vi "TC to PGSQL.vi"(8 "error in (no error)":errorcluster, 11 "TC Cluster":T1) -> (0 "error out":errorcluster)   [LabVIEW 2016]
uses:
  Typedefs/TC-cluster.ctl
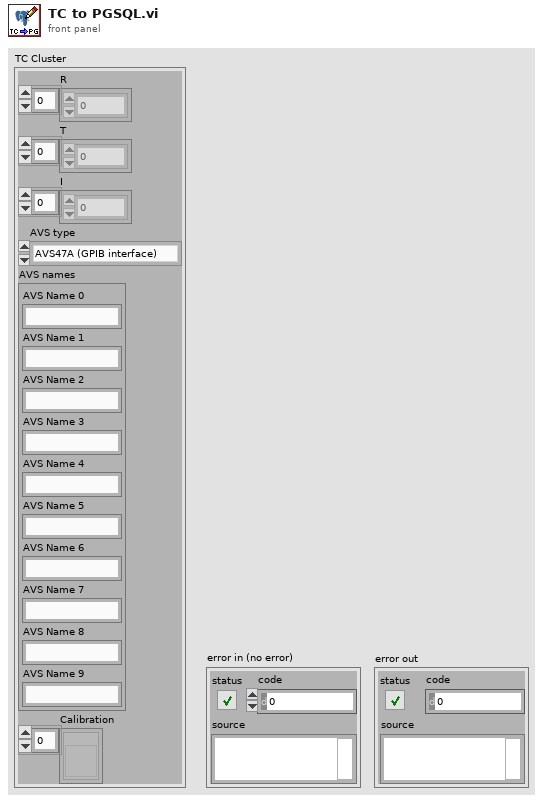
[diagram p1: front panel]
types:
  T1 = typedef "TC-cluster.ctl" = cluster{"R":dbl[], "T":dbl[], "I":dbl[], "AVS type":enum16{"AVS47A (GPIB interface)", "AVS47B (RS232 interface)", "AVS48", "AVS Emulation", "Impedance Bridge", "Disabled"}, "AVS names":cluster{"AVS Name 0":string, "AVS Name 1":string, "AVS Name 2":string, "AVS Name 3":string, "AVS Name 4":string, "AVS Name 5":string, "AVS Name 6":string, "AVS Name 7":string, "AVS Name 8":string, "AVS Name 9":string}, "Calibration":refnum<vi>[]}
  T2 = enum16{"AVS47A (GPIB interface)", "AVS47B (RS232 interface)", "AVS48", "AVS Emulation", "Impedance Bridge", "Disabled"}
  T3 = cluster{"AVS Name 0":string, "AVS Name 1":string, "AVS Name 2":string, "AVS Name 3":string, "AVS Name 4":string, "AVS Name 5":string, "AVS Name 6":string, "AVS Name 7":string, "AVS Name 8":string, "AVS Name 9":string}
  T4 = enum16{"CF", "CF_Z_Bridge", "MNK", "MNK_Z_Bridge"}
  T5 = cluster{"[0]":string, "[1]":string, "[2]":string, "[3]":string, "[4]":string, "[5]":string, "[6]":string, "[7]":string, "[8]":string, "[9]":string}
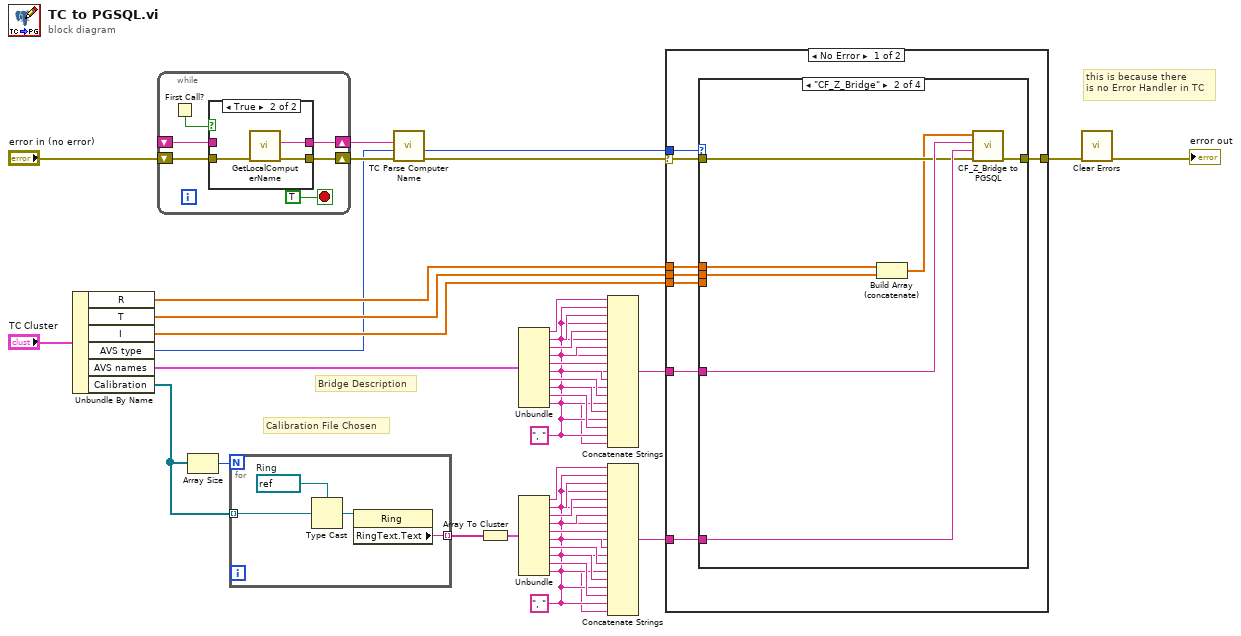
[diagram p0: block diagram]
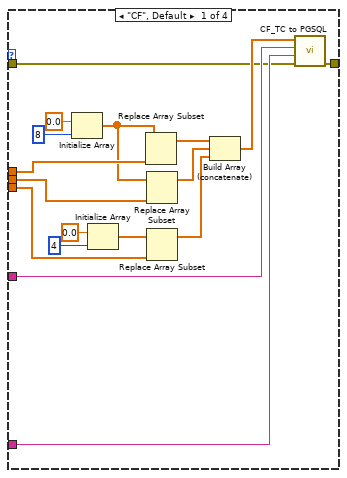
[diagram p3: hidden frame]
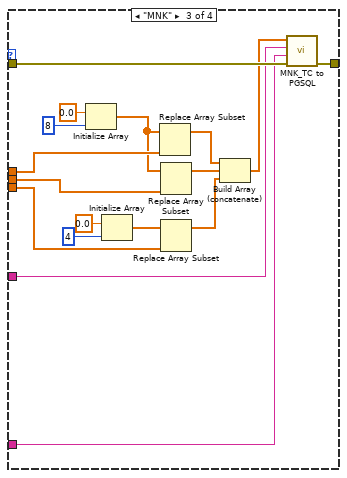
[diagram p4: hidden frame]
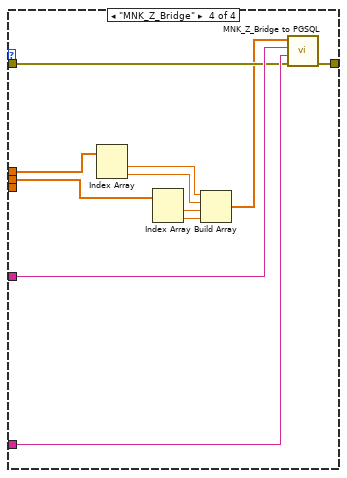
[diagram p5: hidden frame]
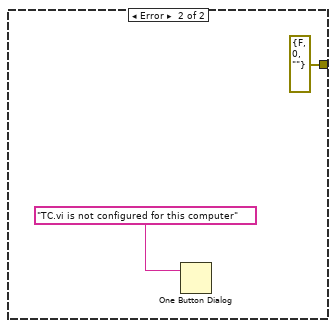
[diagram p6: hidden frame]
diagram:
  w18 = ", " ("string")
  w32 = ", " ("string")
  # "this is because there\nis no Error Handler in TC"
  # "Bridge Description"
  # "Calibration File Chosen"
  n1 = Unbundle By Name("TC Cluster") -> ("R"=w9:dbl[], "T"=w8:dbl[], "I"=w7:dbl[], "AVS type"=w4:T2, "AVS names"=w6:T3, "Calibration"=w5:refnum<vi>[])
  n2 = while {
    shift-right: [w46] -> w12
    shift-left: "error in (no error)" -> [w43]
    shift-right: [w47] -> w3
    shift-left: _ -> [w42]
    stop <- TRUE stop-if-true
    n3 = First Call?() -> (First Call?: T/F=w45:bool)
    n4 = case shown="True" w45 {
      tunnel: [w49 w52] -> w47
      tunnel: [w48 w51] -> w46
      tunnel: w43 -> [w48 w50]
      tunnel: w42 -> [w49 _]
      frame False {
      }
      frame True {
        n5 = call "GetLocalComputerName.vi"("error in (no error)"=w50) -> ("error out"=w51:errorcluster, "Name"=w52:string)  [unwired: 8 in, 1 out]
      }
    }
  }
  n6 = Array Size(array=w5) -> (size(s)=w29:i32)
  n7 = for {
    N: w29 -> [_]
    tunnel: w5 -> [w56] mode=indexing
    tunnel: [w53] -> w28 mode=indexing
    w55 = refnum<vi> refnum  # Ring
    n8 = Type Cast(type=w55, x=w56) -> (*(type *) &x=w54:refnum<vi>)
    n9 = property class="Ring"(reference=w54) -> ("RingText.Text"=w53:string)  [unwired: 1 in, 2 out]
  }
  n10 = call "TC Parse Computer Name.vi"("error in (no error)"=w12, "AVS type"=w4, "computer name"=w3) -> ("error out"=w13:errorcluster, "AVS Type"=w14:T4)  [unwired: 7 in]
  n11 = Array To Cluster(array=w28) -> (cluster=w16:T5)
  n12 = Unbundle(w6) -> ("AVS Name 0"=w41:string, "AVS Name 1"=w40:string, "AVS Name 2"=w39:string, "AVS Name 3"=w38:string, "AVS Name 4"=w37:string, "AVS Name 5"=w36:string, "AVS Name 6"=w35:string, "AVS Name 7"=w34:string, "AVS Name 8"=w33:string, "AVS Name 9"=w31:string)
  n13 = Unbundle(w16) -> ("[0]"=w27:string, "[1]"=w26:string, "[2]"=w25:string, "[3]"=w24:string, "[4]"=w23:string, "[5]"=w22:string, "[6]"=w21:string, "[7]"=w20:string, "[8]"=w19:string, "[9]"=w17:string)
  n14 = Concatenate Strings(w41, w32, w40, w32, w39, w32, w38, w32, w37, w32, w36, w32, w35, w32, w34, w32, w33, w32, w31) -> (w30:string)
  n15 = Concatenate Strings(w27, w18, w26, w18, w25, w18, w24, w18, w23, w18, w22, w18, w21, w18, w20, w18, w19, w18, w17) -> (w15:string)
  n16 = case shown="No Error" w13 {
    selector: w13 -> [w58 _]
    tunnel: w30 -> [w64 _]
    tunnel: w15 -> [w63 _]
    tunnel: w14 -> [w62 _]
    tunnel: w9 -> [w61 _]
    tunnel: w8 -> [w60 _]
    tunnel: w7 -> [w59 _]
    tunnel: [w57 errorcluster {"status"=FALSE, "code"=0, "source"=""} ("error out")] -> w2
    frame No Error {
      n17 = case shown="\"CF_Z_Bridge\"" w62 {
        tunnel: w61 -> [w67 w88 w94 w108]
        tunnel: w60 -> [w65 w87 w93 w106]
        tunnel: w59 -> [w68 _ w92 _]
        tunnel: w64 -> [w81 w86 w102 w112]
        tunnel: w63 -> [w80 w85 w103 w111]
        tunnel: w58 -> [w77 w84 w105 w110]
        tunnel: [w78 w83 w104 w109] -> w57
        frame "CF", Default {
          n18 = Initialize Array(0.0 ("element"), 8 ("dimension size")) -> (w66:dbl[])
          n19 = Initialize Array(0.0 ("element"), 4 ("dimension size")) -> (w70:dbl[])
          n20 = Replace Array Subset(array=w66, new element=w67) -> (w74:dbl[])  [unwired: 1 in]
          n21 = Replace Array Subset(array=w66, new element=w65) -> (w73:dbl[])  [unwired: 1 in]
          n22 = Replace Array Subset(array=w70, new element=w68) -> (w69:dbl[])  [unwired: 1 in]
          n23 = Build Array (concatenate)(w74, w73, w69) -> (w79:dbl[])
          n24 = call "CF_TC to PGSQL.vi"("error in (no error)"=w77, "calibration string"=w80, "description string"=w81, "dbl"=w79) -> ("error out"=w78:errorcluster)  [unwired: 7 in]
        }
        frame "CF_Z_Bridge" {
          n25 = Build Array (concatenate)(w88, w87) -> (w82:dbl[])
          n26 = call "CF_Z_Bridge to PGSQL.vi"("error in (no error)"=w84, "calibration string"=w85, "description string"=w86, "dbl"=w82) -> ("error out"=w83:errorcluster)  [unwired: 7 in]
        }
        frame "MNK" {
          n27 = Initialize Array(0.0 ("element"), 8 ("dimension size")) -> (w89:dbl[])
          n28 = Initialize Array(0.0 ("element"), 4 ("dimension size")) -> (w96:dbl[])
          n29 = Replace Array Subset(array=w89, new element=w94) -> (w100:dbl[])  [unwired: 1 in]
          n30 = Replace Array Subset(array=w89, new element=w93) -> (w99:dbl[])  [unwired: 1 in]
          n31 = Replace Array Subset(array=w96, new element=w92) -> (w95:dbl[])  [unwired: 1 in]
          n32 = Build Array (concatenate)(w100, w99, w95) -> (w91:dbl[])
          n33 = call "MNK_TC to PGSQL.vi"("error in (no error)"=w105, "calibration string"=w103, "description string"=w102, "dbl"=w91) -> ("error out"=w104:errorcluster)  [unwired: 7 in]
        }
        frame "MNK_Z_Bridge" {
          n34 = Index Array(array=w108) -> (element #1=w116:dbl, element #2=w115:dbl)  [unwired: 2 in]
          n35 = Index Array(array=w106) -> (element #1=w114:dbl, element #2=w113:dbl)  [unwired: 2 in]
          n36 = Build Array(w116, w115, w114, w113) -> (w107:dbl[])
          n37 = call "MNK_Z_Bridge to PGSQL.vi"("error in (no error)"=w110, "calibration string"=w111, "description string"=w112, "dbl"=w107) -> ("error out"=w109:errorcluster)  [unwired: 7 in]
        }
      }
    }
    frame Error {
      n38 = One Button Dialog(message="TC.vi is not configured for this computer" ("URL")) -> ()  [unwired: 1 in, 1 out]
    }
  }
  n39 = call <vilib>:"Clear Errors.vi"("error in (no error)"=w2) -> ("error out"=→"error out":errorcluster)  [unwired: 5 in, 1 out]
